vi "Module ID.vi"(11 "HTTP Manager in":refnum<class "HTTP Manager.lvclass">) -> (2 "Module ID":string)   [LabVIEW 2020, in "Volatus.lvlib" / "HTTP Manager.lvclass"]
uses:
  HTTP Manager.lvclass
  HTTP Manager.lvclass/HTTP Manager.ctl
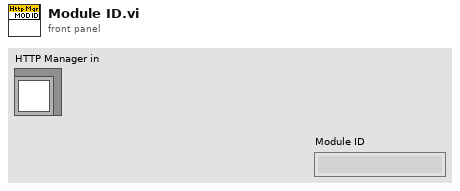
[diagram p1: front panel]
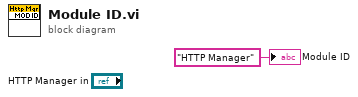
[diagram p0: block diagram]
diagram:
  "Module ID" <- "HTTP Manager" ("Module ID")
